vi "niFpgaUnitDelayTemplate.vi"(0 "input":fxp<+/-,16,16>, 1 "reset":bool, 7 "initial condition":fxp<+/-,16,16>) -> (4 "output":fxp<+/-,16,16>)   [LabVIEW 2017]
doc: "Delays the input value for one cycle. The data type you wire to <B>input</B> determines the <B>output</B> data type."
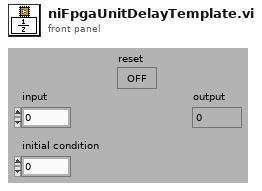
[diagram p1: front panel]
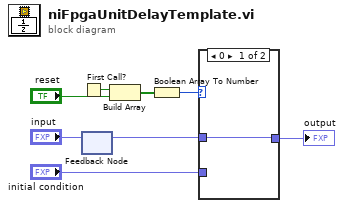
[diagram p0: block diagram]
diagram:
  n1 = First Call?() -> (First Call?: T/F=w4:bool)
  n2 = feedback-in #1("input") -> ()
  n3 = feedback #1() -> (w5:fxp<+/-,16,16>)  [unwired: 1 in]
  n4 = Build Array(w4, "reset") -> (w2:bool[])
  n5 = Boolean Array To Number(Boolean array=w2) -> (number=w1:u8)
  n6 = case shown="0" w1 {
    tunnel: [w9 w10] -> w6
    tunnel: w5 -> [w9 _]
    tunnel: "initial condition" -> [_ w10]
    frame 0 {
    }
    frame Default {
    }
  }
  "output" <- w6
